vi "Nystroem.vi"(8 "error in":errorcluster caption="entrée d'erreur", 11 "Nystroem":T1={"kernel"="rbf", "gamma"="None", "coef0"="None", "degree"="None", "kernel_params"="None", "n_components"=100, "random_state"=-1} {"random_state" min=-1}) -> (0 "error out":errorcluster caption="sortie d'erreur", 3 "Nystroem.lvclass":refnum<class "Nystroem.lvclass">)   [LabVIEW 2020]
doc: "Approximate a kernel map using a subset of the training data.\n\nConstructs an approximate feature map for an arbitrary kernel using a subset of the data as basis.\n\nParameters :\n\n- kernel : string or callable, default=”rbf”\nKernel map to be approximated. A callable should accept two arguments and the keyword arguments passed to this object as kernel_params, and should return a floating point number.\n\n- gamma : float, default=None\nGamma parameter for the RBF, laplacian, polynomial, exponential chi2 and sigmoid kernels. Interpretation of the default value is left to the kernel; see the documentation for sklearn.metrics.pairwise. Ignored by other kernels.\n\n- coef0 : float, default=None\nZero coefficient for polynomial and sigmoid kernels. Ignored by other kernels.\n\n- degree : float, default=None\nDegree of the polynomial kernel. Ignored by other kernels.\n\n- kernel_params : mapping of string to any, optional\nAdditional parameters (keyword arguments) for kernel function passed as callable object.\n\n- n_components : int\nNumber of features to construct. How many data points will be used to construct the mapping.\n\n- random_state : int, RandomState instance or None, optional (default=None=-1)\nPseudo-random number generator to control the uniform sampling without replacement of n_components of the training data to construct the basis kernel. Pass an int for reproducible output across multiple function calls.\n\n\nMethods :\n\n- Fit : Fit estimator to data. Samples a subset of training points, computes kernel on these and computes normalization matrix.\n\nParameters : X : array-like of shape (n_samples, n_features)\nTraining data.\n\n- Fit Transform : Fit to data, then transform it. Fits transformer to X and y with optional parameters fit_params and returns a transformed version of X.\n\nParameters : X : {array-like, sparse matrix, dataframe} of shape (n_samples, n_features)\n y : ndarray of shape (n_samples,), default=None\n Target values.\n\nReturns : X_new : ndarray array of shape (n_samples, n_features_new)\n Transformed array.\n\n\n- Transform : Apply feature map to X. Computes an approximate feature map using the kernel between some training points and X.\n\nParameters : X : array-like of shape (n_samples, n_features)\n Data to transform.\n\nReturns : X_transformed : array, shape=(n_samples, n_components)\n Transformed data."
uses:
  Nystroem.lvclass
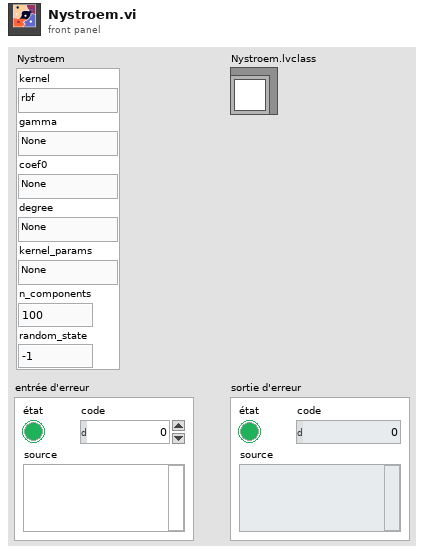
[diagram p1: front panel]
types:
  T1 = cluster{"kernel":string, "gamma":string, "coef0":string, "degree":string, "kernel_params":string, "n_components":i32, "random_state":i32}
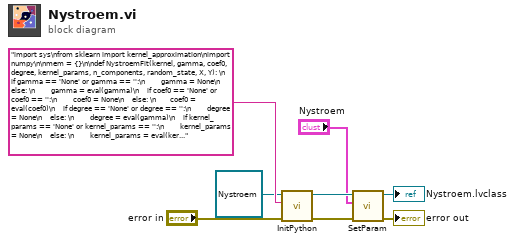
[diagram p0: block diagram]
diagram:
  n1 = call-dynamic "InitPython.vi"("error in (no error)"="error in", "Python Instruction"="import sys\nfrom sklearn import kernel_approximation\nimport numpy\n\nmem = {}\n\ndef NystroemFit(kernel, gamma, coef0, degree, kernel_params, n_components, random_state, X, Y): \n    if gamma == 'None' or gamma == '':\n        gamma = None\n    else: \n        gamma = eval(gamma)\n    if coef0 == 'None' or coef0 == '':\n        coef0 = None\n    else: \n       coef0 = eval(coef0)\n    if degree == 'None' or degree == '':\n        degree = None\n    else: \n        degree = eval(gamma)\n    if kernel_params == 'None' or kernel_params == '':\n        kernel_params = None\n    else: \n        kernel_params = eval(kernel_params)\n    if random_state == -1:\n        random_state = None\n    X = eval(X)\n    if Y == '':\n        Y = None\n    else:\n        Y = eval(Y)\n    try:\n        Nystroem = kernel_approximation.Nystroem(kernel, gamma, coef0, degree, kernel_params, n_components, random_state).fit(X, Y)\n        mem['FitNystroem'] = Nystroem\n        return str('OK')\n    except:\n        erreur = sys.exc_info()\n        typerr = u\"%s\" % (erreur[0])\n        typerr = typerr[typerr.find(\"'\")+1:typerr.rfind(\"'\")]\n        msgerr = u\"%s\" % (erreur[1])\n        message = str('/!\\\\ {0} : {1}'. format(typerr,msgerr))\n        return message \n\ndef NystroemFitTransform(kernel, gamma, coef0, degree, kernel_params, n_components, random_state, X, Y):\n    if gamma == 'None' or gamma == '':\n        gamma = None\n    else: \n        gamma = eval(gamma)\n    if coef0 == 'None' or coef0 == '':\n        coef0 = None\n    else: \n       coef0 = eval(coef0)\n    if degree == 'None' or degree == '':\n        degree = None\n    else: \n        degree = eval(gamma)\n    if kernel_params == 'None' or kernel_params == '':\n        kernel_params = None\n    else: \n        kernel_params = eval(kernel_params)\n    if random_state == -1:\n        random_state = None\n    X = eval(X)\n    if Y == '':\n        Y = None\n    else:\n        Y = eval(Y)\n    try:\n        Nystroem = kernel_approximation.Nystroem(kernel, gamma, coef0, degree, kernel_params, n_components, random_state).fit_transform(X, Y)\n        Nystroem = Nystroem.tolist()\n        return str(Nystroem)\n    except:\n        erreur = sys.exc_info()\n        typerr = u\"%s\" % (erreur[0])\n        typerr = typerr[typerr.find(\"'\")+1:typerr.rfind(\"'\")]\n        msgerr = u\"%s\" % (erreur[1])\n        message = str('/!\\\\ {0} : {1}'. format(typerr,msgerr))\n        return message \n    \n\ndef NystroemTransform(kernel, gamma, coef0, degree, kernel_params, n_components, random_state, X, Y):\n    if gamma == 'None' or gamma == '':\n        gamma = None\n    else: \n        gamma = eval(gamma)\n    if coef0 == 'None' or coef0 == '':\n        coef0 = None\n    else: \n       coef0 = eval(coef0)\n    if degree == 'None' or degree == '':\n        degree = None\n    else: \n        degree = eval(gamma)\n    if kernel_params == 'None' or kernel_params == '':\n        kernel_params = None\n    else: \n        kernel_params = eval(kernel_params)\n    if random_state == -1:\n        random_state = None\n    X = eval(X)\n    if Y == '':\n        Y = None\n    else:\n        Y = eval(Y)\n    try:\n        Nystroem = mem['FitNystroem'].transform(X, Y)\n        Nystroem = Nystroem.tolist()\n        return str(Nystroem)\n    except:\n        erreur = sys.exc_info()\n        typerr = u\"%s\" % (erreur[0])\n        typerr = typerr[typerr.find(\"'\")+1:typerr.rfind(\"'\")]\n        msgerr = u\"%s\" % (erreur[1])\n        message = str('/!\\\\ {0} : {1}'. format(typerr,msgerr))\n        return message", "Scikit-learn en entrée"=refnum<class "Nystroem.lvclass"> refnum ("Nystroem.lvclass")) -> ("error out"=w3:errorcluster, "Scikit-learn en sortie"=w5:refnum<class "Nystroem.lvclass">)  [unwired: 7 in]
  n2 = call-dynamic "SetParam.vi"("error in (no error)"=w3, "Nystroem"="Nystroem", "Nystroem.lvclass"=w5) -> ("error in (no error)"=→"error out":errorcluster, "Nystroem.lvclass"=→"Nystroem.lvclass":refnum<class "Nystroem.lvclass">)  [unwired: 7 in]
